vi "measure down hole pressure and save to csv file.vi"(0 "Path in":refnum<vi>, 1 "Descriptions Reference":refnum<vi>, 2 "Input Variables and Slopes Reference":refnum<vi>, 5 "Sensor Reference":refnum<vi>, 7 "Zero Pressure Reference 5":refnum<vi>, 9 "Record DTW File":bool, 11 "error in (no error)":errorcluster, 12 "Array in":refnum<k24>[](array[refnum]), 13 "Input Variables and Slopes":T1 {"Height of Sample Box" format="%.2f"; "Reservoir Pressure" format="%.2f"; "Flow Offset" format="%.2f"; "String Pot Offset" format="%.2f"; "Aux 3 Offset" format="%.2f"; "Aux 2 Offset" format="%.2f"; "Aux 1 Offset" format="%.2f"; "Aux 3 Slope" format="%.2f"; "Aux 2 Slope" format="%.2f"; "Aux 1 Slope" format="%.2f"; "Up Hole  Pressure Offset" format="%.2f"; "DH Pressure Offset" format="%.2f"; "DH Pressure Trans Slope" format="%.2f"; "Atmospheric Pressure" format="%.2f"; "Depth to Water Table" format="%.2f"; "Up Hole Pressure Slope" format="%.2f"; "Flow Slope" format="%.2f"; "String Pot Slope" format="%.2f"; "Total Volume" format="%.2f"}) -> (4 "DTW path 2":path, 6 "Array out":refnum<k24>[](array[refnum]), 8 "Down Hole Pressure\n(ft/H20)":dbl format="%.2f", 10 "DHT Pressure (V)":dbl format="%.2f", 15 "error out":errorcluster)   [LabVIEW 2016]
uses:
  Control 2.ctl
  C:/Cascade-lv16-64/builds/Waterloo Main Program/cascade/data/ULx_LV.dll
  builds/Waterloo Main Program/cascade/data/ULx_LV.dll
  Kpro Globals.vi
  <vilib>/Utility/file.llb/Write Delimited Spreadsheet (DBL).vi
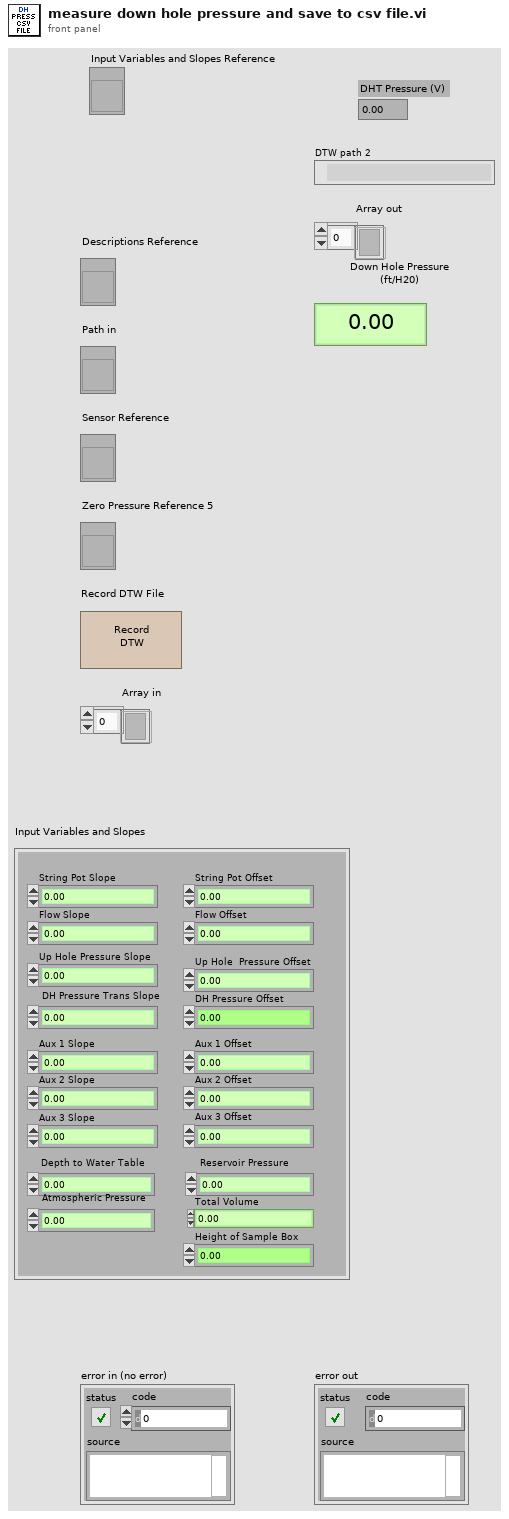
[diagram p1: front panel]
types:
  T1 = typedef "Control 2.ctl" = cluster{"Total Volume":dbl, "String Pot Slope":dbl, "Flow Slope":dbl, "Up Hole Pressure Slope":dbl, "Depth to Water Table":dbl, "Atmospheric Pressure":dbl, "DH Pressure Trans Slope":dbl, "DH Pressure Offset":dbl, "Up Hole  Pressure Offset":dbl, "Aux 1 Slope":dbl, "Aux 2 Slope":dbl, "Aux 3 Slope":dbl, "Aux 1 Offset":dbl, "Aux 2 Offset":dbl, "Aux 3 Offset":dbl, "String Pot Offset":dbl, "Flow Offset":dbl, "Reservoir Pressure":dbl, "Height of Sample Box":dbl}
  T2 = typedef "MCC DAQ Readings.ctl" = cluster{"Uphole Pressure":dbl, "Flow":dbl, "Downhole Pressure":dbl, "Top String Pot":dbl, "String Pot":dbl, "Aux 1":dbl, "Aux 2":dbl, "Aux 3":dbl, "9V Monitor":dbl}
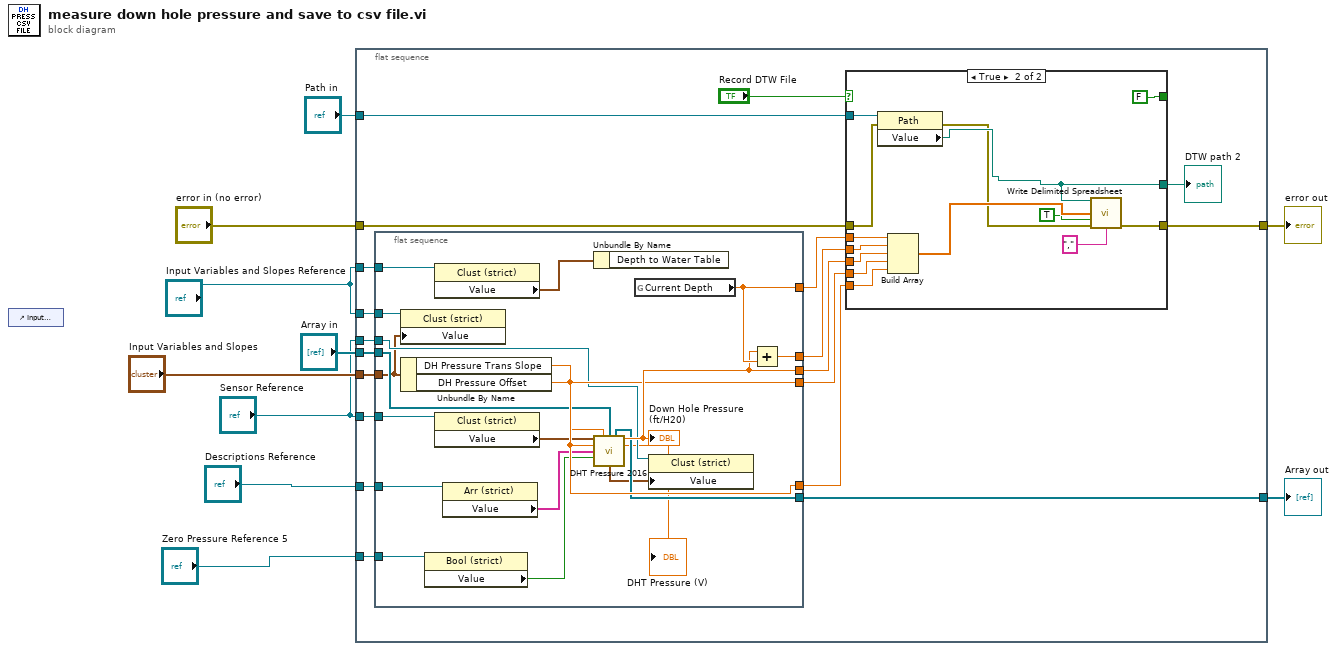
[diagram p0: block diagram]
diagram:
  n1 = control-ref of="Input Variables and Slopes"() -> ()  [unwired: 1 out]
  n2 = flat-sequence {
    tunnel: "Array in" -> [w23]
    tunnel: [w22] -> w7
    tunnel: "Input Variables and Slopes" -> [w21]
    tunnel: "error in (no error)" -> [w20]
    tunnel: [w19] -> w10
    tunnel: "Path in" -> [w17]
    tunnel: "Input Variables and Slopes Reference" -> [w16]
    tunnel: "Descriptions Reference" -> [w15]
    tunnel: "Sensor Reference" -> [w14]
    tunnel: "Sensor Reference" -> [w13]
    tunnel: "Zero Pressure Reference 5" -> [w12]
    tunnel: "Input Variables and Slopes Reference" -> [w11]
    frame #0 {
      n3 = flat-sequence {
        tunnel: [w49] -> w29
        tunnel: [w48] -> w27
        tunnel: [w47] -> w26
        tunnel: [w46] -> w25
        tunnel: [w45] -> w24
        tunnel: w23 -> [w44]
        tunnel: [w43] -> w22
        tunnel: w21 -> [w31]
        tunnel: w16 -> [w37]
        tunnel: w15 -> [w36]
        tunnel: w14 -> [w35]
        tunnel: w13 -> [w34]
        tunnel: w12 -> [w33]
        tunnel: w11 -> [w32]
        frame #0 {
          n4 = property class="Clust (strict)"(reference=w37, "Value"=w31) -> ()  [unwired: 1 in, 2 out]
          n5 = Unbundle By Name(w31) -> ("DH Pressure Trans Slope"=w46:dbl, "DH Pressure Offset"=w45:dbl)
          n6 = property class="Bool (strict)"(reference=w33) -> ("Value"=w39:bool)  [unwired: 1 in, 2 out]
          n7 = property class="Clust (strict)"(reference=w32) -> ("Value"=w38:T1)  [unwired: 1 in, 2 out]
          n8 = property class="Clust (strict)"(reference=w35) -> ("Value"=w41:T2)  [unwired: 1 in, 2 out]
          n9 = property class="Arr (strict)"(reference=w36) -> ("Value"=w42:string[])  [unwired: 1 in, 2 out]
          n10 = Unbundle By Name(w38) -> ()  [unwired: 1 out]
          n11 = call "DHT Pressure 2016.vi"("Sensor Cluster"=w41, "DHT Pressure Offset"=w45, "Array in"=w44, "DHT Pressure \nSlope"=w46, "Descriptions"=w42, "Zero Pressure\n(F = leave as is)"=w39) -> ("Array out"=w43:refnum<k24>[], "DHT Pressure (ft/H20)"=w47:dbl, "DHT Pressure (V)"=→"DHT Pressure (V)":dbl, "Sensor Cluster 2"=w40:T2)  [unwired: 6 in]
          "Down Hole Pressure\n(ft/H20)" <- w47
          n12 = global read "Kpro Globals.vi" "Current Depth"() -> (w49:sgl)
          n13 = property class="Clust (strict)"(reference=w34, "Value"=w40) -> ()  [unwired: 1 in, 2 out]
          n14 = Add(x=w47, y=w49) -> (x+y=w48:dbl)
        }
      }
      n15 = case shown="True" "Record DTW File" {
        selector: "Record DTW File" -> [w51 _]
        tunnel: [w51 FALSE ("Boolean")] -> _
        tunnel: w27 -> [_ w61]
        tunnel: w29 -> [_ w62]
        tunnel: w24 -> [_ w59]
        tunnel: w26 -> [_ w60]
        tunnel: w25 -> [_ w58]
        tunnel: w20 -> [w50 w53]
        tunnel: [w50 w57] -> w19
        tunnel: [_ w54] -> w18
        tunnel: w17 -> [_ w55]
        frame False {
        }
        frame True {
          n16 = property class="Path"(reference=w55, error in=w53) -> (error out=w52:errorcluster, "Value"=w54:path)  [unwired: 1 out]
          n17 = Build Array(w62, w61, w60, w59, w58) -> (w65:dbl[])
          n18 = call-poly <vilib>:"Write Delimited Spreadsheet.vi"("file path (dialog if empty)"=w54, "1D data"=w65, "append to file? (new file:F)"=TRUE, "error in (no error)"=w52, "delimiter (\\t)"="," ("delimiter (\\t)")) -> ("error out"=w57:errorcluster)  [unwired: 9 in, 1 out]
        }
      }
      "DTW path 2" <- w18
    }
  }
  "error out" <- w10
  "Array out" <- w7
